vi "measure_voltage_V2.vi"(0 "VISA resource name":refnum<visa-resource-name>, 11 "error in":errorcluster) -> (4 "VISA resource name out":refnum<visa-resource-name>, 6 "MEASure:VOLTage? CH1 Chart":dbl(graph), 8 "MEASure:VOLTage? CH2 Chart":dbl(graph), 10 "output Array":dbl[](array[numeric]), 15 "error out":errorcluster)   [LabVIEW 2020]
uses:
  controls/SCPI_enum.ctl
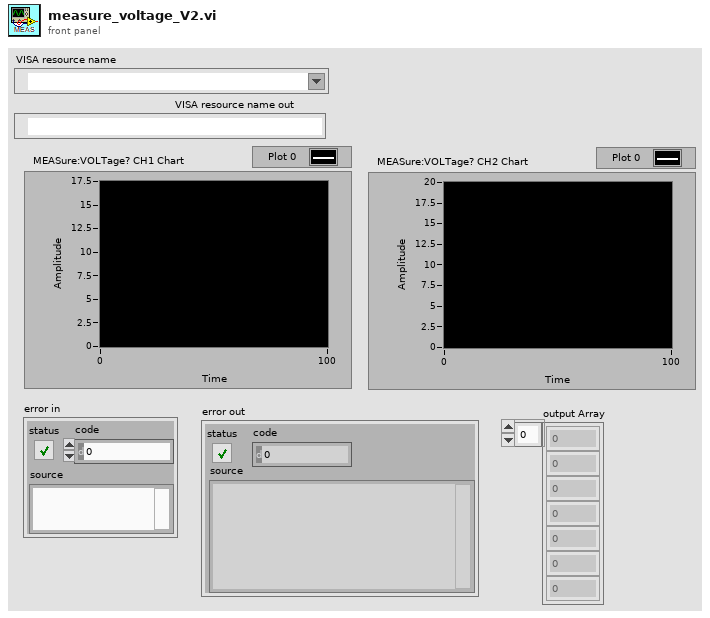
[diagram p1: front panel]
types:
  T1 = typedef "SCPI_enum.ctl" = u16
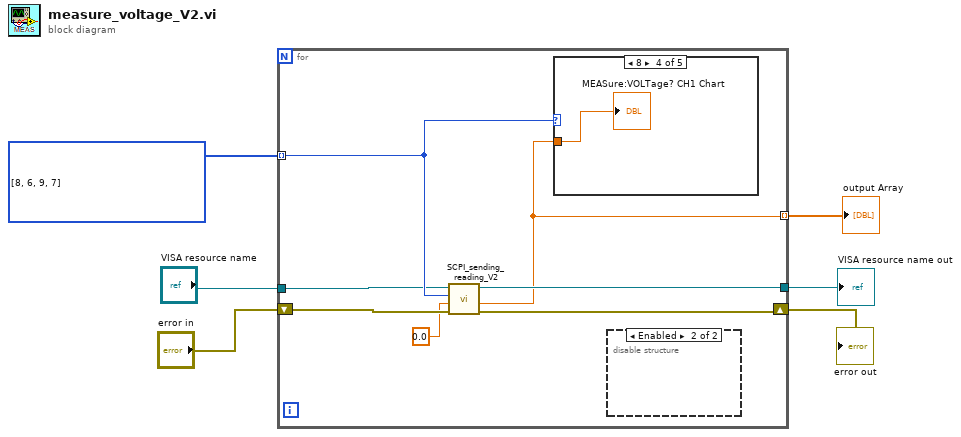
[diagram p0: block diagram]
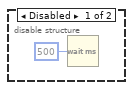
[diagram p2: hidden frame]
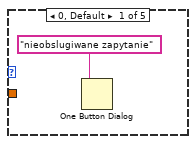
[diagram p3: hidden frame]
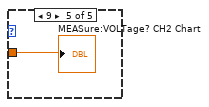
[diagram p6: hidden frame]
diagram:
  w6 = T1[] [8, 6, 9, 7] items=["*IDN?", "*SAV 1", "*RCL 1", "INSTTrument CH1", "INSTTrument CH2", "INSTrument?", "MEASure:CURRent? CH1", "MEASure:CURRent? CH2", "MEASure:VOLTage? CH1", "MEASure:VOLTage? CH2", "MEASure:POWEr? CH1", "MEASure:POWEr? CH2", "CH1:CURRent?", "CH2:CURRent?", "CH1:VOLTage? ", "CH2:VOLTage? ", "OUTPut CH1,ON", "OUTPut CH1,OFF", "OUTPut CH2,ON", "OUTPut CH2,OFF", "OUTPut CH3,ON", "OUTPut CH3,OFF", "OUTPut:TRACK 0", "OUTPut:TRACK 1", "OUTPut:TRACK 2", "OUTPut:WAVE CH1,ON", "OUTPut:WAVE CH1,OFF", "OUTPut:WAVE CH2,ON", "OUTPut:WAVE CH2,OFF", "CH1:VOLTage", "CH2:VOLTage", "CH1:CURRent", "CH2:CURRent"]
  n1 = for {
    tunnel: w6 -> [w10] mode=indexing
    tunnel: [w12] -> w2
    shift-right: [w11] -> w4
    shift-left: "error in" -> [w13]
    tunnel: "VISA resource name" -> [w9]
    tunnel: [w8] -> w1 mode=indexing
    n2 = call "SCPI_sending_reading_V2.vi"("error in (no error)"=w13, "Numeric entrece"=0.0, "SCIPI"=w10, "VISA"=w9) -> ("error out"=w11:errorcluster, "read numeric value"=w8:dbl, "VISA resource name out"=w12:refnum<visa-resource-name>)  [unwired: 1 out]
    n3 = case shown="8" w10 {
      tunnel: w8 -> [_ _ _ w16 w17]
      frame 0, Default {
        n4 = One Button Dialog(message="nieobslugiwane zapytanie") -> ()  [unwired: 1 in, 1 out]
      }
      frame 6 {
      }
      frame 7 {
      }
      frame 8 {
        "MEASure:VOLTage? CH1 Chart" <- w16
      }
      frame 9 {
        "MEASure:VOLTage? CH2 Chart" <- w17
      }
    }
    n5 = disable-structure shown="Enabled" {
      frame Disabled {
        n6 = Wait (ms)(milliseconds to wait=u32 500) -> ()  [unwired: 1 out]
      }
      frame Enabled {
      }
    }
  }
  "error out" <- w4
  "VISA resource name out" <- w2
  "output Array" <- w1
